vi "App Version.vi"() -> (2 "App Version":string)   [LabVIEW 2020, in "Volatus.lvlib" / "App.lvclass"]
uses:
  App.lvclass
  App.lvclass/App.ctl
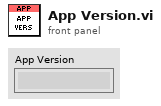
[diagram p1: front panel]
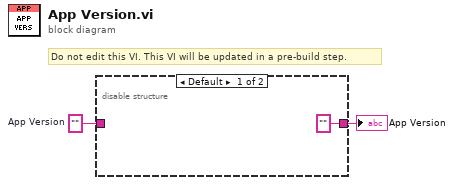
[diagram p0: block diagram]
diagram:
  w2 = ""  # App Version
  # "Do not edit this VI. This VI will be updated in a pre-build step."
  n1 = disable-structure shown="Default" {
    disable-tunnel: w2 -> [_ w4]
    disable-tunnel: ["" ("App Version") w4] -> w1
    frame condition #0 (active) {
    }
    frame condition #1 {
    }
  }
  "App Version" <- w1
